vi "Settings Dialog.vi"(8 "error in (no error)":errorcluster, 11 "Settings in":T12={"Hardware Configuration"={"VISA resource name"="", "DAQ Type"=0, "Channel 1"={"Acquiring"=FALSE, "Enabled"=FALSE, "Terminal configuration"=32767, "Range"=0, "Coupling"=0}, "Channel 2"={"Acquiring"=FALSE, "Enabled"=FALSE, "Terminal configuration"=0, "Range"=0, "Coupling"=0}, "Timing"={"Sample Time [Time Units]"=0, "Actual Sample Time [s]"=0.0, "Samples per Iteration"=0, "Sample Clock Source"=0, "Time Units"=0, "t0"=timestamp(0 s since 1904-01-01)}, "PS Parameters"={"PS handle"=0, "PS Max_adc"=32767, "PS Enabled Array"=[], "PS Device Info"={"Driver Version"="", "USB Version"="", "Hardware"="", "Variant"="", "Batch and Serial"="", "Cal Date"="", "Kernel Version"="", "Digital HW Version"="", "Analogue HW Version"="", "Firmware 1"="", "Firmware 2"="", "MSO"=FALSE, "Number of Channels"=0}, "Channel 1 Buffer"=refnum, "Channel 2 Buffer"=refnum, "Resolution"=0, "USB Power"=FALSE}, "Trigger"={"Direction"=0, "Threshold [V]"=0.0, "Enabled"=FALSE, "Trigger Source"=0}, "Keithley Parameters"={"Previous End / Current Start"=0, "Quantity"=0}}, "Logging Configuration"={"Log File Base Path"=path "", "TDMS File Reference"=refnum, "Enabled"=FALSE, "Disk cache size"=0}} {"Hardware Configuration"."Keithley Parameters"."Quantity" items=["Current", "Voltage"]; "Hardware Configuration"."Trigger"."Trigger Source" items=["Channel 1"=0, "Channel 2"=1, "Ext."=4]; "Hardware Configuration"."Trigger"."Direction" items=["Falling", "Rising"]; "Hardware Configuration"."PS Parameters"."Resolution" items=["8", "12", "14", "15", "16"]; "Hardware Configuration"."Timing"."Time Units" items=["Seconds"]; "Hardware Configuration"."Timing"."Sample Clock Source" items=["Internal", "External"]; "Hardware Configuration"."Channel 2"."Coupling" items=["AC", "DC"]; "Hardware Configuration"."Channel 2"."Range" items=["0.01", "0.02", "0.05", "0.1", "0.2", "0.5", "1", "2", "5", "10", "20", "50", "100", "1000"]; "Hardware Configuration"."Channel 2"."Terminal configuration" items=["Referenced Single Ended", "Differential"]; "Hardware Configuration"."Channel 1"."Coupling" items=["AC", "DC"]; "Hardware Configuration"."Channel 1"."Range" items=["0.01", "0.02", "0.05", "0.1", "0.2", "0.5", "1", "2", "5", "10", "20", "50", "100", "1000"]; "Hardware Configuration"."Channel 1"."Terminal configuration" items=["Referenced Single Ended", "Differential"]; "Hardware Configuration"."DAQ Type" items=["Simulated", "Tektronics DPO2k/3k/4k", "PicoScope 2000a Series", "Keithley DMM7510", "PicoScope 5000a Series"]}) -> (0 "error out":errorcluster, 1 "Cancelled?":bool, 2 "UI Refresh Needed?":bool, 3 "Settings out":T12={"Hardware Configuration"={"VISA resource name"="", "DAQ Type"=0, "Channel 1"={"Acquiring"=FALSE, "Enabled"=FALSE, "Terminal configuration"=32767, "Range"=0, "Coupling"=0}, "Channel 2"={"Acquiring"=FALSE, "Enabled"=FALSE, "Terminal configuration"=0, "Range"=0, "Coupling"=0}, "Timing"={"Sample Time [Time Units]"=0, "Actual Sample Time [s]"=0.0, "Samples per Iteration"=0, "Sample Clock Source"=0, "Time Units"=0, "t0"=timestamp(0 s since 1904-01-01)}, "PS Parameters"={"PS handle"=0, "PS Max_adc"=32767, "PS Enabled Array"=[], "PS Device Info"={"Driver Version"="", "USB Version"="", "Hardware"="", "Variant"="", "Batch and Serial"="", "Cal Date"="", "Kernel Version"="", "Digital HW Version"="", "Analogue HW Version"="", "Firmware 1"="", "Firmware 2"="", "MSO"=FALSE, "Number of Channels"=0}, "Channel 1 Buffer"=refnum, "Channel 2 Buffer"=refnum, "Resolution"=0, "USB Power"=FALSE}, "Trigger"={"Direction"=0, "Threshold [V]"=0.0, "Enabled"=FALSE, "Trigger Source"=0}, "Keithley Parameters"={"Previous End / Current Start"=0, "Quantity"=0}}, "Logging Configuration"={"Log File Base Path"=path "", "TDMS File Reference"=refnum, "Enabled"=FALSE, "Disk cache size"=0}} {"Hardware Configuration"."Keithley Parameters"."Quantity" items=["Current", "Voltage"]; "Hardware Configuration"."Trigger"."Trigger Source" items=["Channel 1"=0, "Channel 2"=1, "Ext."=4]; "Hardware Configuration"."Trigger"."Direction" items=["Falling", "Rising"]; "Hardware Configuration"."PS Parameters"."Resolution" items=["8", "12", "14", "15", "16"]; "Hardware Configuration"."Timing"."Time Units" items=["Seconds"]; "Hardware Configuration"."Timing"."Sample Clock Source" items=["Internal", "External"]; "Hardware Configuration"."Channel 2"."Coupling" items=["AC", "DC"]; "Hardware Configuration"."Channel 2"."Range" items=["0.01", "0.02", "0.05", "0.1", "0.2", "0.5", "1", "2", "5", "10", "20", "50", "100", "1000"]; "Hardware Configuration"."Channel 2"."Terminal configuration" items=["Referenced Single Ended", "Differential"]; "Hardware Configuration"."Channel 1"."Coupling" items=["AC", "DC"]; "Hardware Configuration"."Channel 1"."Range" items=["0.01", "0.02", "0.05", "0.1", "0.2", "0.5", "1", "2", "5", "10", "20", "50", "100", "1000"]; "Hardware Configuration"."Channel 1"."Terminal configuration" items=["Referenced Single Ended", "Differential"]; "Hardware Configuration"."DAQ Type" items=["Simulated", "Tektronics DPO2k/3k/4k", "PicoScope 2000a Series", "Keithley DMM7510", "PicoScope 5000a Series"]})   [LabVIEW 2016, in "Settings.lvlib"]
doc: "Dialog for selecting user specified settings."
uses:
  Settings.lvlib
  Settings.ctl
  Acquisition/Hardware Configuration.ctl
  Acquisition/Signal Type.ctl
  Terminal Configuration.ctl
  Range.ctl
  Coupling.ctl
  Sampling Clock Source.ctl
  Time Units.ctl
  Resolution.ctl
  Trigger Direction.ctl
  Trigger Source.ctl
  Quantity.ctl
  Logging/Logging Configuration.ctl
  Physical Connection.ctl
  <vilib>/Utility/xml.llb/Write to XML File(string).vi
  Acquisition/Acquisition.lvlib
  Logging/Logging.lvlib
panel:
  in  "Quantity":T1=1 items=["Current", "Voltage"]
  in  "USB Powered":bool
  in  "Resolution":T2 items=["8", "12", "14", "15", "16"]
  in  "Coupling":T3=1 items=["AC", "DC"]
  in  "Coupling":T3=1 items=["AC", "DC"]
  in  "Time Unit":T4=4 items=["ns"=2, "us"=3, "ms"=4, "s"=5]
  in  "Tab Control":enum32{"Disabled", "Analog", "Digital"}(tab)
  in  "Direction":T5 items=["Either"=0, "Rising"=3, "Falling"=4]
  in  "Threshold [V]":dbl
  in  "Trigger Source":T6 items=["Channel 1"=0, "Channel 2"=1, "External"=4]
  in  "On/Off":bool=TRUE
  in  "Range":T7 items=["10 u"=50, "100 u"=51, "1 m"=52, "10 m"=0, "20 m"=1, "50 m"=2, "100 m"=3, "200 m"=4, "500 m"=5, "1"=6, "2"=7, "3"=53, "5"=8, "10"=9, "20"=10, "50"=11, "100"=12, "700"=90, "1000"=13]
  in  "Range":T7 items=["10 u"=50, "100 u"=51, "1 m"=52, "10 m"=0, "20 m"=1, "50 m"=2, "100 m"=3, "200 m"=4, "500 m"=5, "1"=6, "2"=7, "3"=53, "5"=8, "10"=9, "20"=10, "50"=11, "100"=12, "700"=90, "1000"=13]
  out "Samples per Iteration":dbl
  out "Actual Samping Time":dbl
  in  "Sampling Time":u32=1 min=1
  in  "Sampling Clock Source":T8 items=["Internal", "External"]
  out "Acquiring":bool
  out "Acquiring":bool
  in  "Terminal configuration":T9 items=["Referenced Single Ended", "Differential"]
  in  "Physical connection":T10 items=["Disabled", "Channel 1", "Channel 2"]
  in  "Terminal configuration":T9 items=["Referenced Single Ended", "Differential"]
  in  "Physical connection":T10 items=["Disabled", "Channel 1", "Channel 2"]
  in  "VISA resource name":refnum<visa-resource-name>
  in  "Log File Path":path
  in  "DAQ Type":T11 items=["Simulated", "Tektronics DPO2k/3k/4k", "PicoScope 2000a Series", "Keithley DMM7510", "PicoScope 5000a Series"]
  in  "Cancel Button":bool
  in  "OK Button":bool
  # "Non visible portion of dialog (needed for connector pane)."
  # "General Settings"
  # "Timing Settings"
  # "Channel Settings (Signal 1)"
  # "Trigger Settings"
  # "Channel Settings (Signal 2)"
  # "Logging"
  # "To configure and use a start trigger you must select\nthe specific tab. Not all hardware supports triggering.\nRefer to your device documentation for more info"
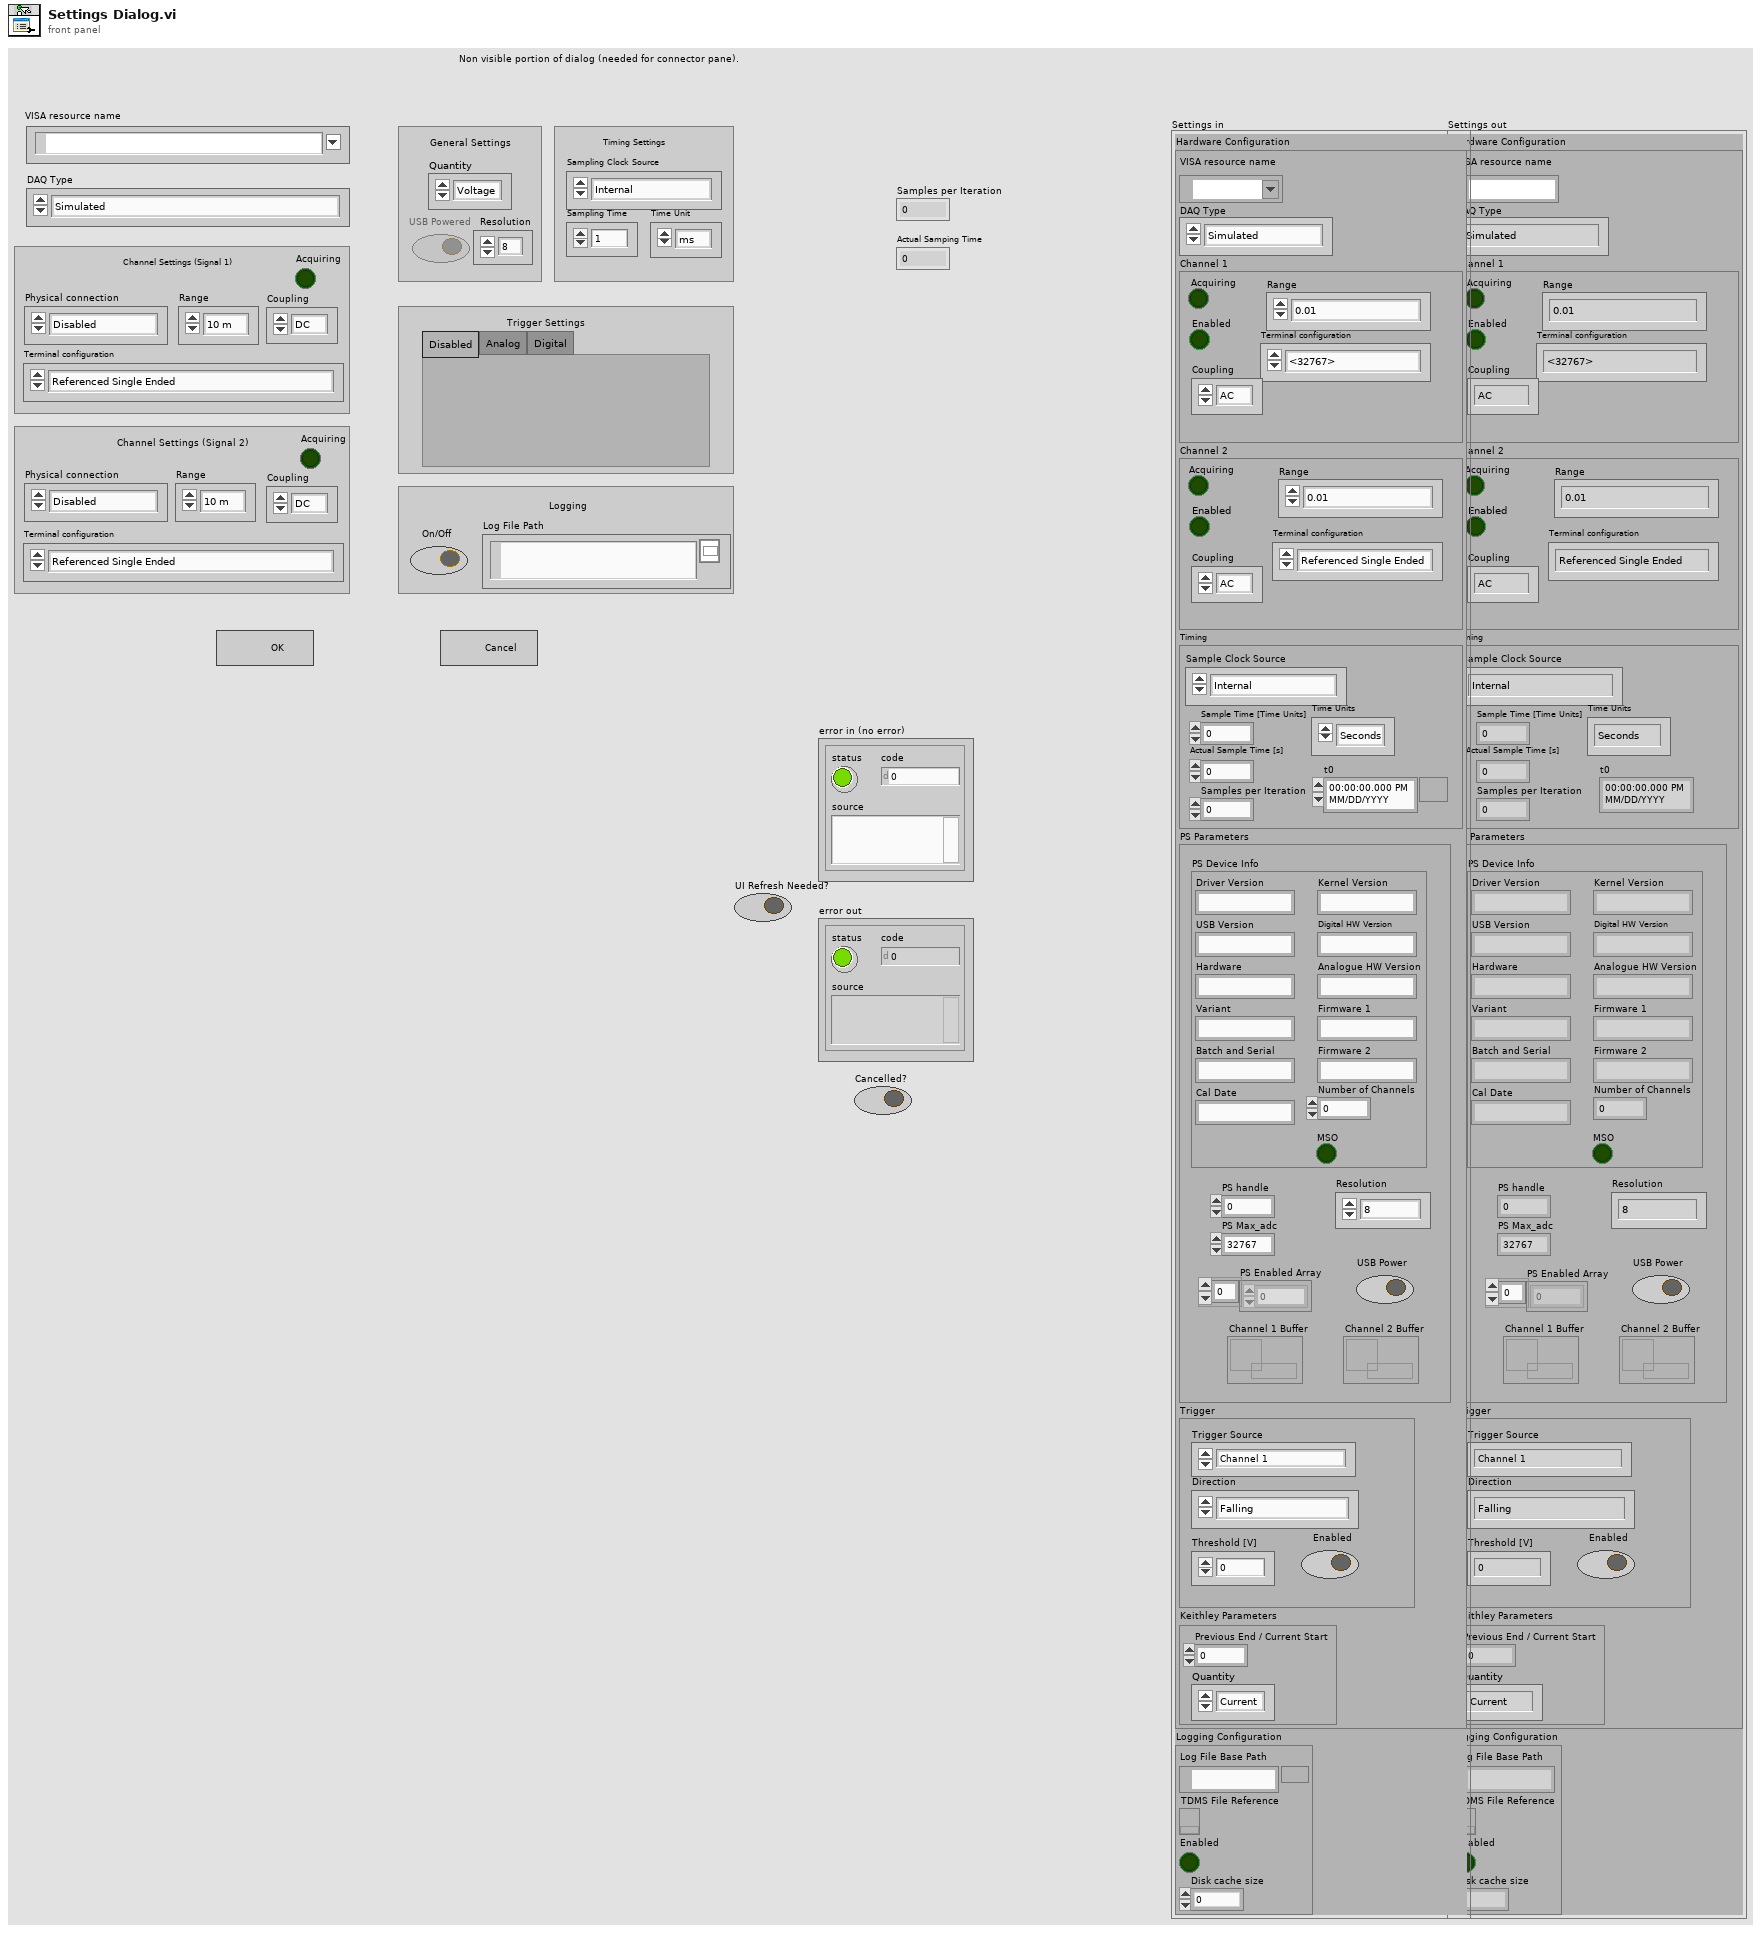
[diagram p1: front panel]
types:
  T1 = typedef "Settings.lvlib/Quantity.ctl" = u16
  T2 = typedef "Settings.lvlib/Resolution.ctl" = i32
  T3 = typedef "Settings.lvlib/Coupling.ctl" = i16
  T4 = typedef "Settings.lvlib/Time Units.ctl" = u32
  T5 = typedef "Settings.lvlib/Trigger Direction.ctl" = u16
  T6 = typedef "Settings.lvlib/Trigger Source.ctl" = u16
  T7 = typedef "Settings.lvlib/Range.ctl" = u16
  T8 = typedef "Settings.lvlib/Sampling Clock Source.ctl" = u16
  T9 = typedef "Settings.lvlib/Terminal Configuration.ctl" = u16
  T10 = typedef "Settings.lvlib/Physical Connection.ctl" = u16
  T11 = typedef "Acquisition.lvlib/Signal Type.ctl" = u16
  T12 = typedef "Settings.lvlib/Settings.ctl" = cluster{"Hardware Configuration":T13, "Logging Configuration":T14}
  T13 = typedef "Acquisition.lvlib/Hardware Configuration.ctl" = cluster{"VISA resource name":refnum<visa-resource-name>, "DAQ Type":T11, "Channel 1":cluster{"Acquiring":bool, "Enabled":bool, "Terminal configuration":T9, "Range":T7, "Coupling":T3}, "Channel 2":cluster{"Acquiring":bool, "Enabled":bool, "Terminal configuration":T9, "Range":T7, "Coupling":T3}, "Timing":cluster{"Sample Time [Time Units]":u32, "Actual Sample Time [s]":dbl, "Samples per Iteration":u32, "Sample Clock Source":T8, "Time Units":T4, "t0":timestamp}, "PS Parameters":cluster{"PS handle":i16, "PS Max_adc":i16, "PS Enabled Array":i16[], "PS Device Info":cluster{"Driver Version":string, "USB Version":string, "Hardware":string, "Variant":string, "Batch and Serial":string, "Cal Date":string, "Kernel Version":string, "Digital HW Version":string, "Analogue HW Version":string, "Firmware 1":string, "Firmware 2":string, "MSO":bool, "Number of Channels":i16}, "Channel 1 Buffer":refnum<data-value>, "Channel 2 Buffer":refnum<data-value>, "Resolution":T2, "USB Power":bool}, "Trigger":cluster{"Direction":T5, "Threshold [V]":dbl, "Enabled":bool, "Trigger Source":T6}, "Keithley Parameters":cluster{"Previous End / Current Start":i32, "Quantity":T1}}
  T14 = typedef "Logging.lvlib/Logging Configuration.ctl" = cluster{"Log File Base Path":path, "TDMS File Reference":refnum<k34>, "Enabled":bool, "Disk cache size":u64}
  T15 = enum8{"Enabled", "Disabled", "Disabled and Grayed Out"}
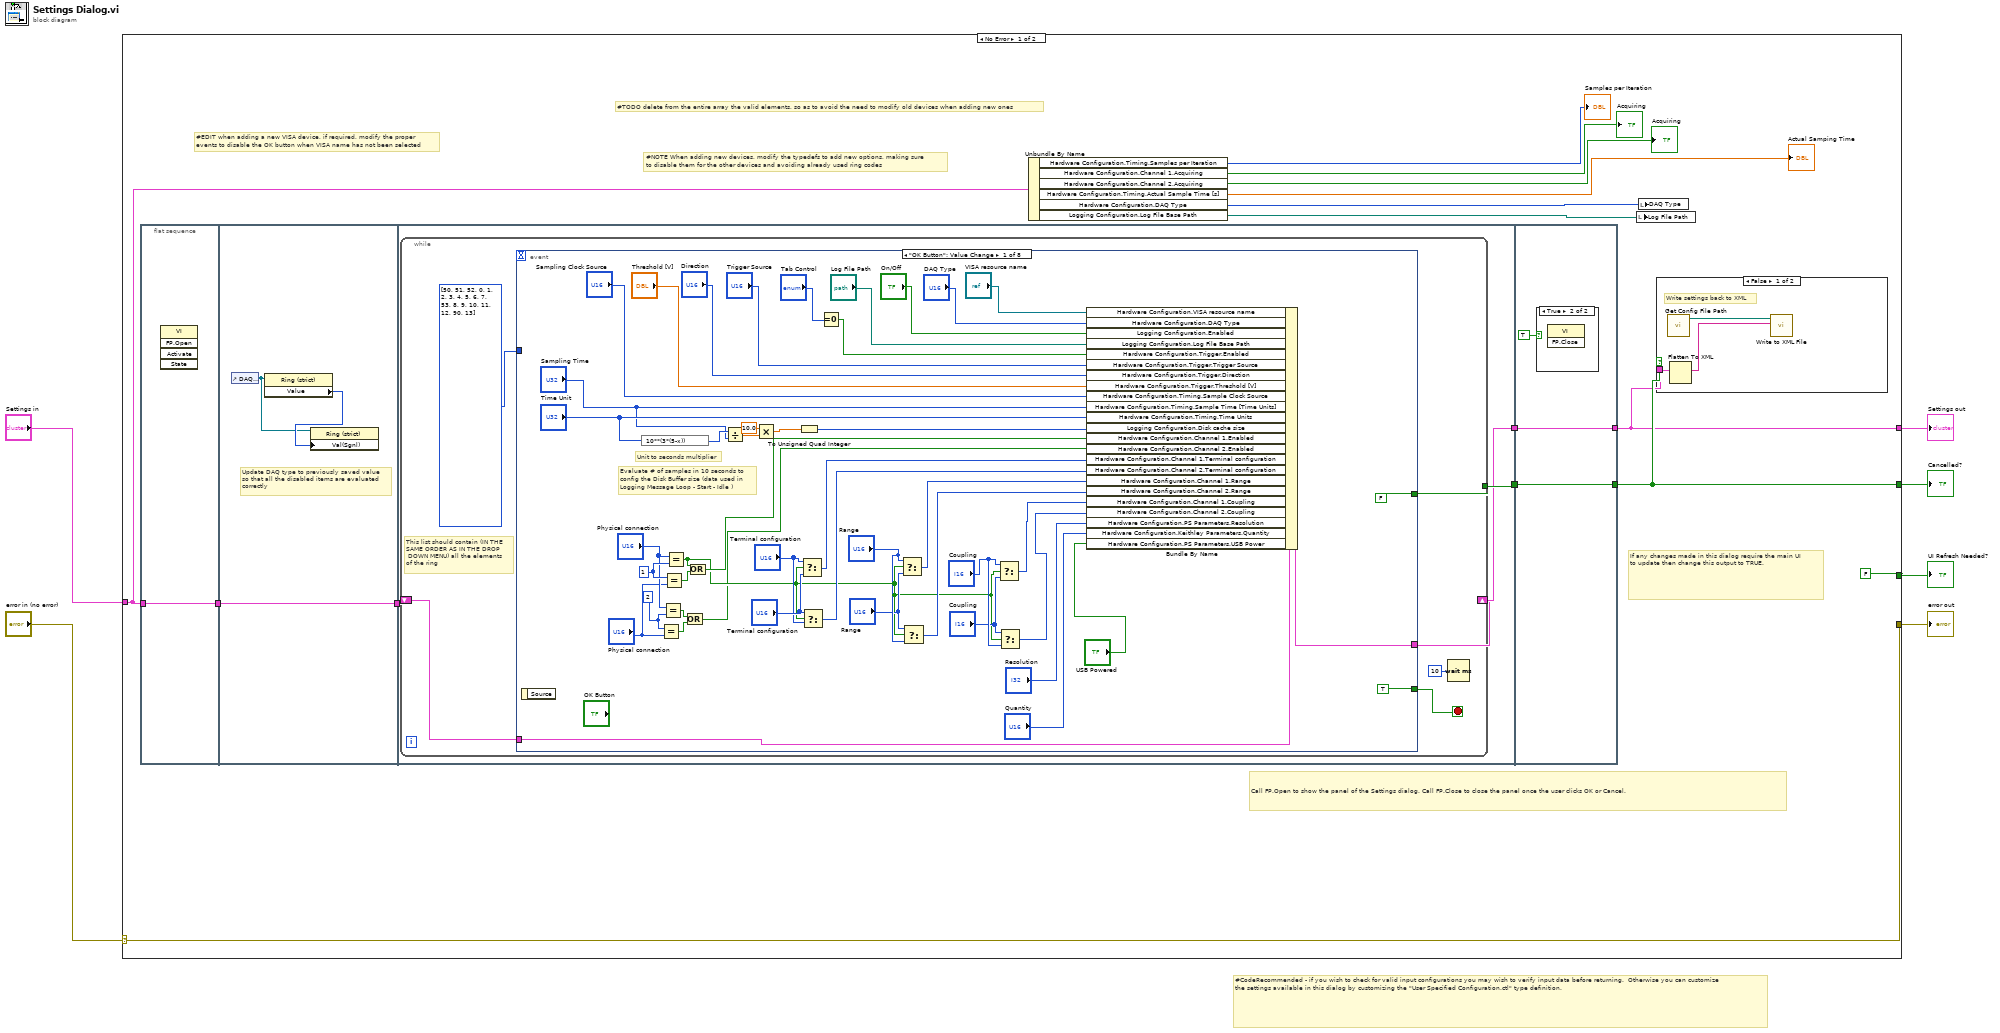
[diagram p0: block diagram]
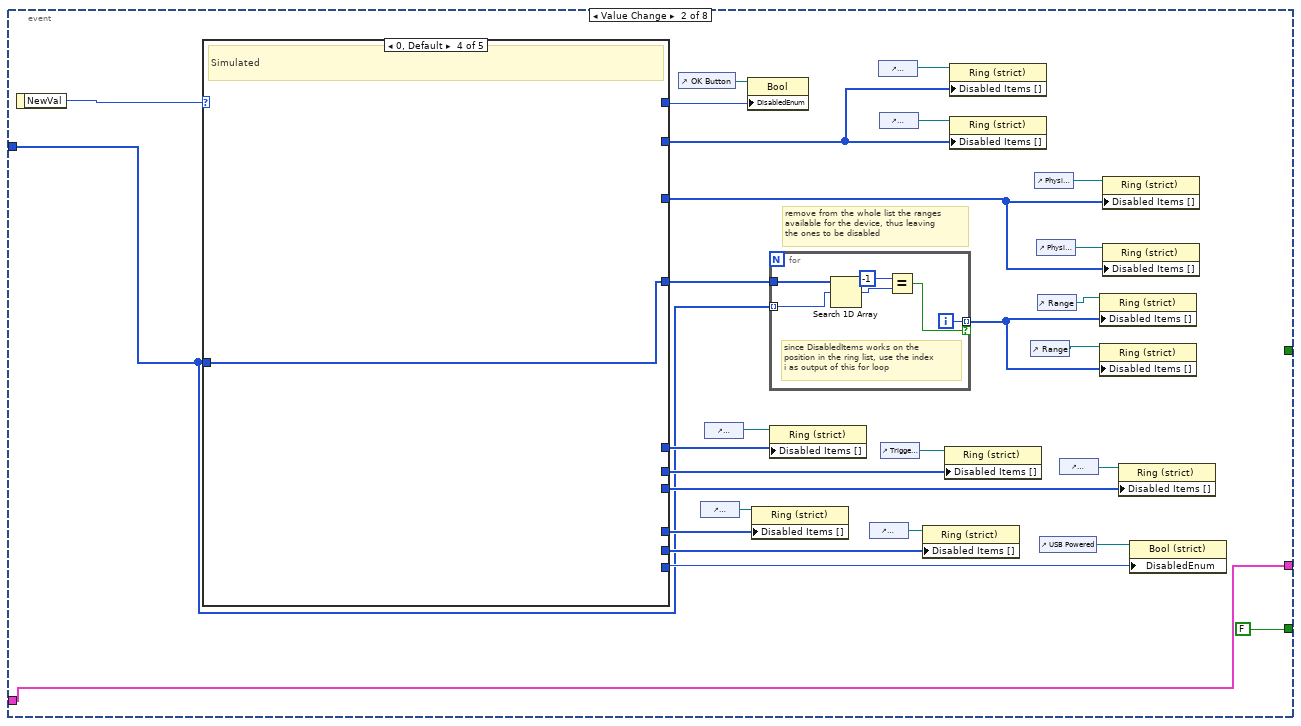
[diagram p2: hidden frame]
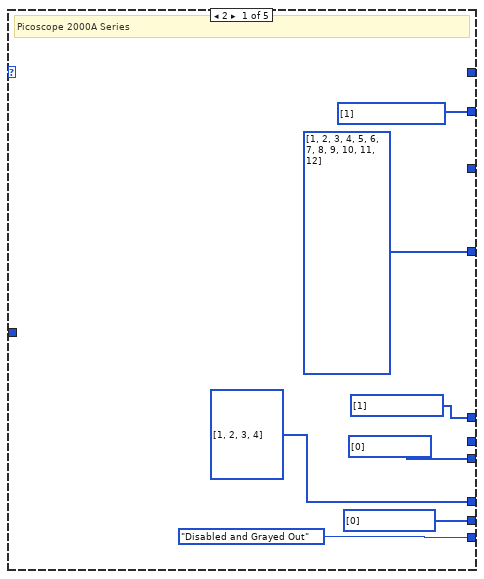
[diagram p3: hidden frame]
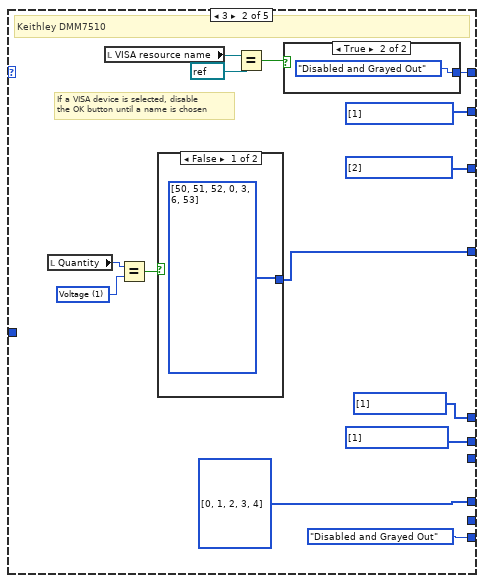
[diagram p4: hidden frame]
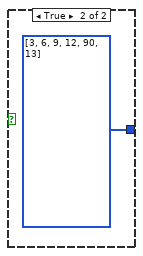
[diagram p5: hidden frame]
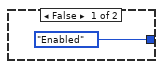
[diagram p6: hidden frame]
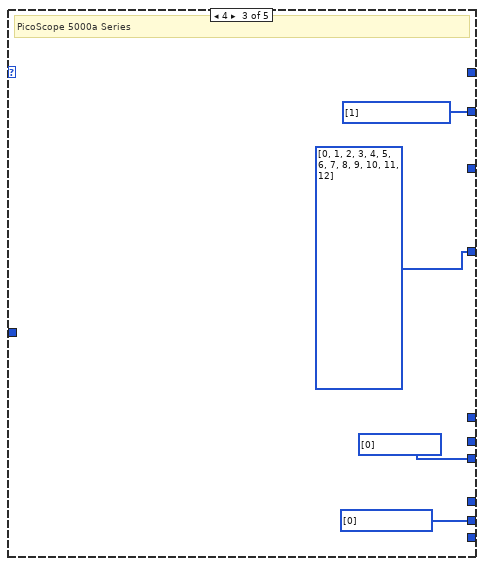
[diagram p7: hidden frame]
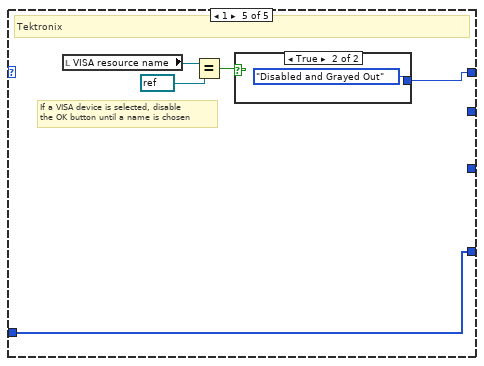
[diagram p8: hidden frame]
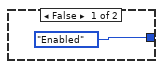
[diagram p9: hidden frame]
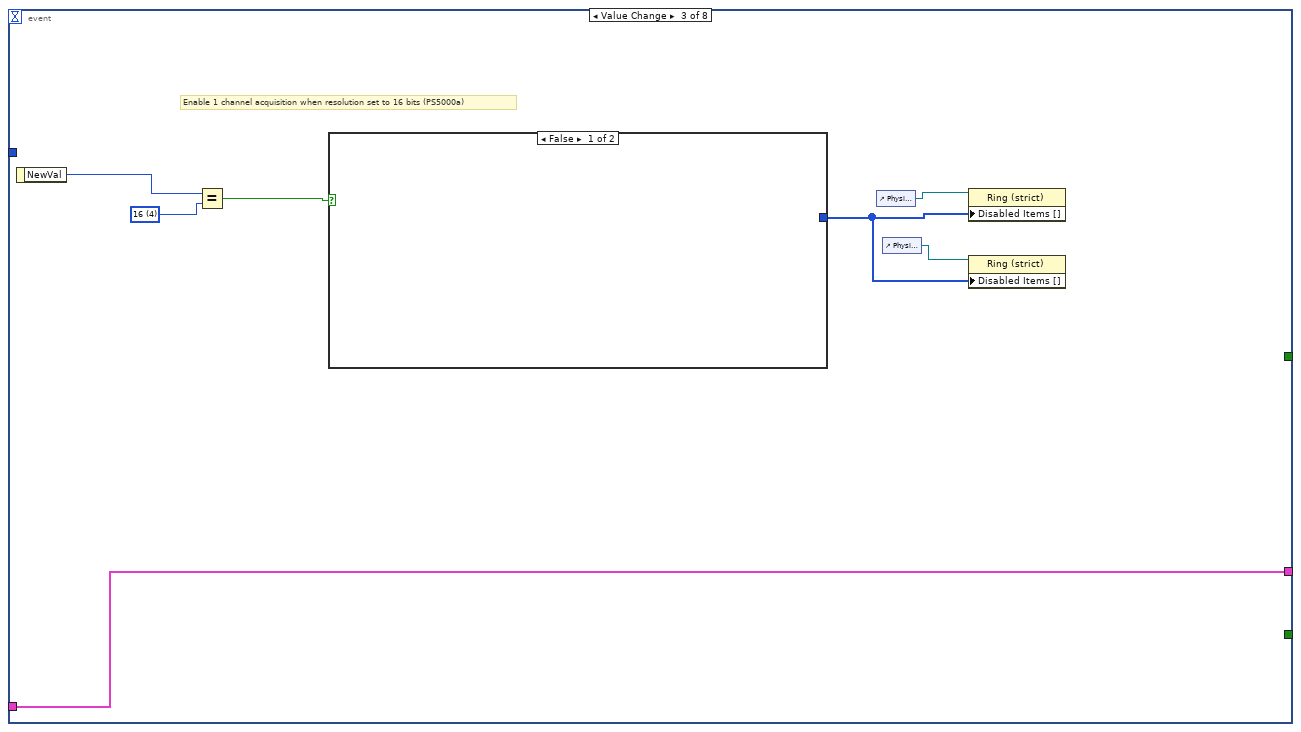
[diagram p10: hidden frame]
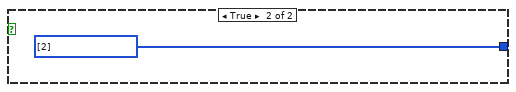
[diagram p11: hidden frame]
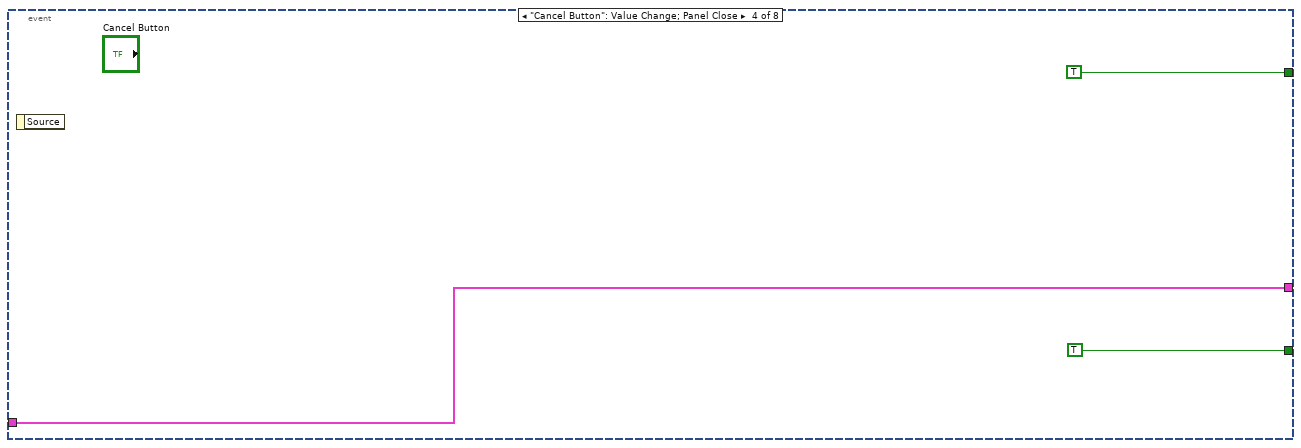
[diagram p12: hidden frame]
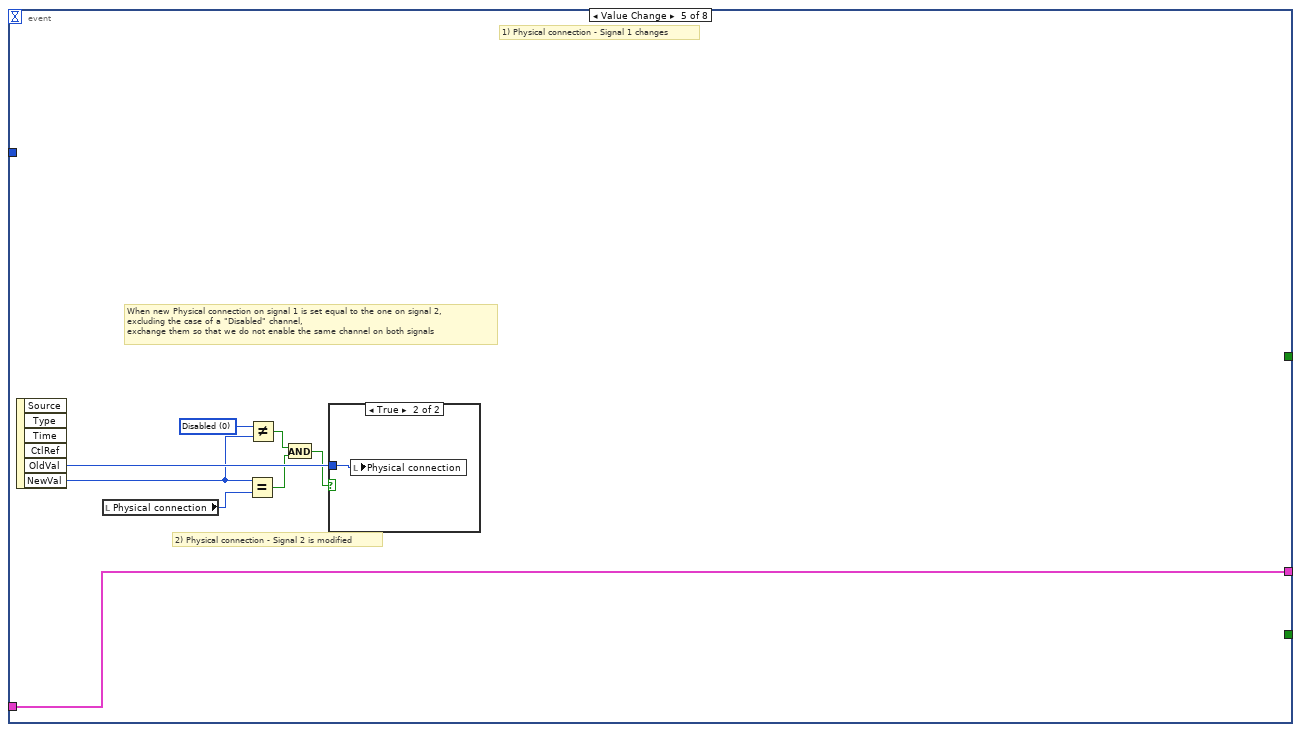
[diagram p13: hidden frame]
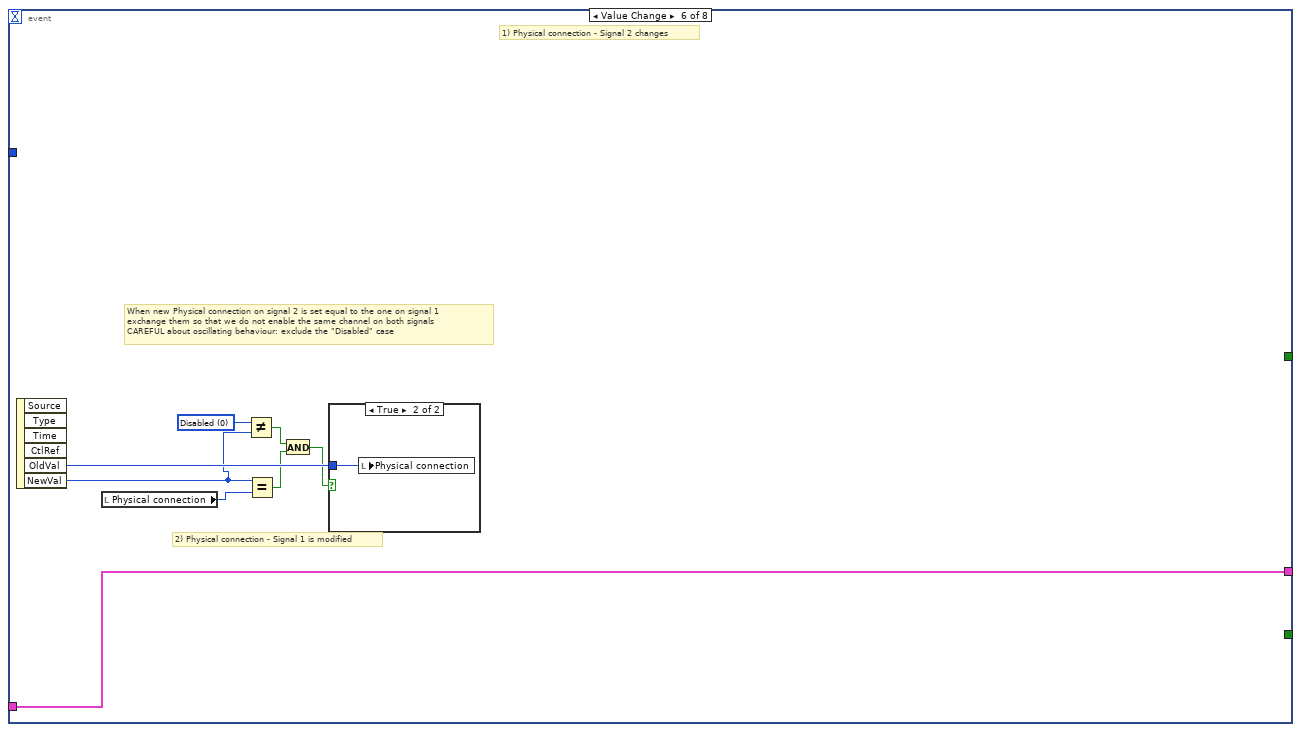
[diagram p15: hidden frame]
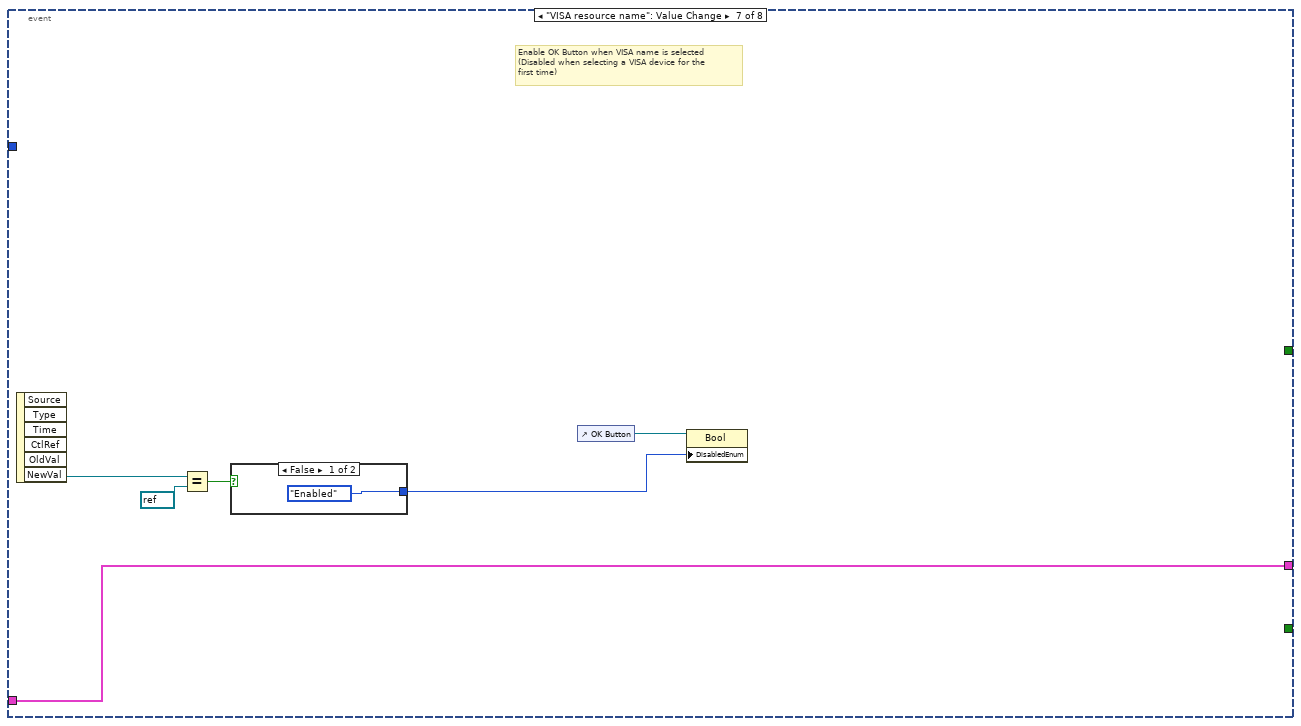
[diagram p17: hidden frame]
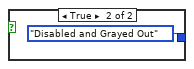
[diagram p18: hidden frame]
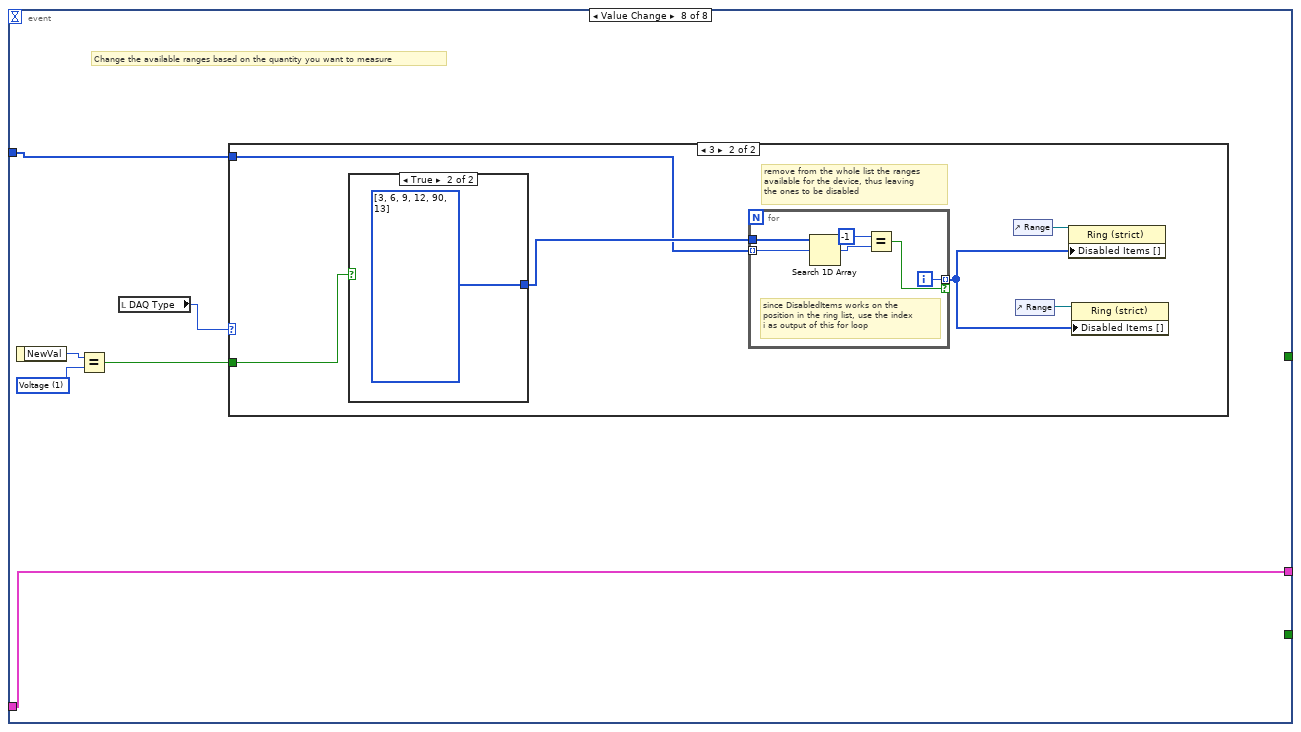
[diagram p19: hidden frame]
diagram:
  # "#CodeRecommended - if you wish to check for valid input configurations you may wish to verify input data before returning.  Otherwise you can customize the settings available in this dialog by customizing the \"User Specified Configuration.ctl\" type definition."
  n1 = case shown="No Error" "error in (no error)" {
    selector: "error in (no error)" -> [w21 w217]
    tunnel: [w21 w217] -> w5
    tunnel: "Settings in" -> [w17 w216]
    tunnel: [w18 w216] -> w3
    tunnel: [FALSE ("UI Refresh Needed?") _] -> w2
    tunnel: [w19 TRUE ("UI Refresh Needed?")] -> w1
    frame No Error {
      # "#EDIT when adding a new VISA device, if required, modify the proper\nevents to disable the OK button when VISA name has not been selected"
      # "#TODO delete from the entire array the valid elements, so as to avoid the need to modify old devices when adding new ones"
      # "#NOTE When adding new devices, modify the typedefs to add new options, making sure\nto disable them for the other devices and avoiding already used ring codes"
      # "Call FP.Open to show the panel of the Settings dialog. Call FP.Close to close the panel once the user clicks OK or Cancel."
      # "If any changes made in this dialog require the main UI to update then change this output to TRUE."
      n2 = flat-sequence {
        tunnel: w17 -> [w22]
        tunnel: [w22] -> w8
        tunnel: w8 -> [w25]
        tunnel: [w25] -> w7
        tunnel: w7 -> [w26]
        tunnel: [w28] -> w14
        tunnel: [w27] -> w13
        tunnel: [w210] -> w18
        tunnel: [w211] -> w19
        tunnel: w14 -> [w211]
        tunnel: w13 -> [w210]
        frame #0 {
          n3 = invoke class="VI" method="FP.Open"() -> ()  [unwired: 5 in, 5 out]
        }
        frame #1 {
          # "Update DAQ type to previously saved value\nso that all the disabled items are evaluated\ncorrectly"
          n4 = control-ref of="DAQ Type"() -> (w23:refnum<vi>)
          n5 = property class="Ring (strict)"(reference=w23) -> ("Value"=w24:T11)  [unwired: 1 in, 2 out]
          n6 = property class="Ring (strict)"(reference=w23, "Val(Sgnl)"=w24) -> ()  [unwired: 1 in, 2 out]
        }
        frame #2 {
          n7 = while {
            tunnel: [w34] -> w28
            shift-right: [w33] -> w27
            shift-left: w26 -> [w32]
            stop <- w31 stop-if-true
            w29 = T7[] [50, 51, 52, 0, 1, 2, 3, 4, 5, 6, 7, 53, 8, 9, 10, 11, 12, 90, 13] items=["10 u"=50, "100 u"=51, "1 m"=52, "10 m"=0, "20 m"=1, "50 m"=2, "100 m"=3, "200 m"=4, "500 m"=5, "1"=6, "2"=7, "3"=53, "5"=8, "10"=9, "20"=10, "50"=11, "100"=12, "700"=90, "1000"=13] ("Range [V]")
            # "This list should contain (IN THE \nSAME ORDER AS IN THE DROP\n DOWN MENU) all the elements \nof the ring"
            n8 = event shown="[0] \"OK Button\": Value Change" {
              selector: _ -> [_ _ _ _ _ _ _ _]
              dyn-events: _ -> [_ _ _ _ _ _ _ _]
              timeout: _ -> [_ _ _ _ _ _ _ _]
              tunnel: [w78 w108 w158 w162 w170 w179 w186 w194] -> w33
              tunnel: w32 -> [w79 w108 w158 w162 w170 w179 w186 w194]
              tunnel: [FALSE ("UI Refresh Needed?") _ _ TRUE ("UI Refresh Needed?") _ _ _ _] -> w34
              tunnel: [TRUE FALSE _ TRUE _ _ _ _] -> w31
              tunnel: w29 -> [_ w81 _ _ _ _ _ w189]
              event "OK Button": Value Change {
                w71 = u16 2 ("x")
                w73 = u16 1 ("x")
                # "Evaluate # of samples in 10 seconds to \nconfig the Disk Buffer size (data used in \nLogging Message Loop - Start - Idle )"
                # "Unit to seconds multiplier"
                n9 = event-data() -> ()  [unwired: 1 in, 1 out]
                n10 = expression code="10**(3*(5-x))"("Time Unit") -> (w40:T4)
                n11 = Equal?(x=w71, y="Physical connection") -> (x = y?=w70:bool)
                n12 = Equal?(x="Physical connection", y=w71) -> (x = y?=w62:bool)
                n13 = Equal?(x=w73, y="Physical connection") -> (x = y?=w72:bool)
                n14 = Equal?(x="Physical connection", y=w73) -> (x = y?=w49:bool)
                n15 = Or(x=w62, y=w70) -> (x .or. y?=w48:bool)
                n16 = Or(x=w49, y=w72) -> (x .or. y?=w59:bool)
                n17 = Divide(x=w40, y="Sampling Time") -> (x/y=w38:dbl)
                n18 = Multiply(x=10.0, y=w38) -> (x*y=w36:dbl)
                n19 = To Unsigned Quad Integer(1:w36) -> (0:w35:u64)
                n20 = Select(t="Terminal configuration", s=w49, f="Terminal configuration") -> (s? t:f=w47:T9)
                n21 = Select(t="Terminal configuration", s=w49, f="Terminal configuration") -> (s? t:f=w65:T9)
                n22 = Equal To 0?(x="Tab Control") -> (x = 0?=w57:bool)
                n23 = Select(t="Range", s=w49, f="Range") -> (s? t:f=w61:T7)
                n24 = Select(t="Range", s=w49, f="Range") -> (s? t:f=w53:T7)
                n25 = Select(t="Coupling", s=w49, f="Coupling") -> (s? t:f=w46:T3)
                n26 = Select(t="Coupling", s=w49, f="Coupling") -> (s? t:f=w45:T3)
                n27 = Bundle By Name(cluster=w79, "Hardware Configuration.VISA resource name"="VISA resource name", "Hardware Configuration.DAQ Type"="DAQ Type", "Logging Configuration.Enabled"="On/Off", "Logging Configuration.Log File Base Path"="Log File Path", "Hardware Configuration.Trigger.Enabled"=w57, "Hardware Configuration.Trigger.Trigger Source"="Trigger Source", "Hardware Configuration.Trigger.Direction"="Direction", "Hardware Configuration.Trigger.Threshold [V]"="Threshold [V]", "Hardware Configuration.Timing.Sample Clock Source"="Sampling Clock Source", "Hardware Configuration.Timing.Sample Time [Time Units]"="Sampling Time", "Hardware Configuration.Timing.Time Units"="Time Unit", "Logging Configuration.Disk cache size"=w35, "Hardware Configuration.Channel 1.Enabled"=w59, "Hardware Configuration.Channel 2.Enabled"=w48, "Hardware Configuration.Channel 1.Terminal configuration"=w47, "Hardware Configuration.Channel 2.Terminal configuration"=w65, "Hardware Configuration.Channel 1.Range"=w61, "Hardware Configuration.Channel 2.Range"=w53, "Hardware Configuration.Channel 1.Coupling"=w46, "Hardware Configuration.Channel 2.Coupling"=w45, "Hardware Configuration.PS Parameters.Resolution"="Resolution", "Hardware Configuration.Keithley Parameters.Quantity"="Quantity", "Hardware Configuration.PS Parameters.USB Power"="USB Powered") -> (w78:T12)
              }
              event Value Change {
                # "remove from the whole list the ranges\navailable for the device, thus leaving \nthe ones to be disabled"
                n28 = event-data() -> ("NewVal"=w107:T11)  [unwired: 1 in]
                n29 = case shown="0, Default" w107 {
                  tunnel: [w121 w135 w143 _ _] -> w103
                  tunnel: [_ w134 _ _ _] -> w100
                  tunnel: [w120 w133 _ _ _] -> w98
                  tunnel: [_ w132 _ _ _] -> w96
                  tunnel: [w119 _ w142 _ _] -> w94
                  tunnel: [w118 w131 _ _ _] -> w92
                  tunnel: [w117 _ w141 _ _] -> w90
                  tunnel: [T15."Disabled and Grayed Out" ("Disabled") T15."Disabled and Grayed Out" ("Disabled") _ _ _] -> w88
                  tunnel: [_ w126 _ _ w146] -> w84
                  tunnel: [w115 w122 w140 w144 w145] -> w82
                  tunnel: w81 -> [_ _ _ w144 w145]
                  frame 2 {
                    w115 = T7[] [1, 2, 3, 4, 5, 6, 7, 8, 9, 10, 11, 12] items=["10 u"=50, "100 u"=51, "1 m"=52, "10 m"=0, "20 m"=1, "50 m"=2, "100 m"=3, "200 m"=4, "500 m"=5, "1"=6, "2"=7, "3"=53, "5"=8, "10"=9, "20"=10, "50"=11, "100"=12, "700"=90, "1000"=13] ("Disabled Items []")
                    w117 = T1[] [0] items=["Current", "Voltage"] ("Disabled Items []")
                    w118 = T2[] [1, 2, 3, 4] items=["8", "12", "14", "15", "16"] ("Disabled Items []")
                    w119 = u16[] [0] items=["Either"=0, "Rising"=3, "Falling"=4] ("Disabled Items []")
                    w120 = u16[] [1] items=["Internal", "External"] ("Disabled Items []")
                    w121 = T9[] [1] items=["Referenced Single Ended", "Differential"] ("Disabled Items []")
                    # "Picoscope 2000A Series"
                  }
                  frame 3 {
                    w124 = T1 1 items=["Current", "Voltage"] ("y")
                    w131 = T2[] [0, 1, 2, 3, 4] items=["8", "12", "14", "15", "16"] ("Disabled Items []")
                    w132 = u16[] [1] items=["Channel 1"=0, "Channel 2"=1, "External"=4] ("Disabled Items []")
                    w133 = u16[] [1] items=["Internal", "External"] ("Disabled Items []")
                    w134 = T10[] [2] items=["Disabled", "Channel 1", "Channel 2"] ("Disabled Items []")
                    w135 = T9[] [1] items=["Referenced Single Ended", "Differential"] ("Disabled Items []")
                    # "If a VISA device is selected, disable\nthe OK button until a name is chosen"
                    # "Keithley DMM7510"
                    n30 = local read "Quantity"() -> (w123:T1)
                    n31 = local read "VISA resource name"() -> (w129:refnum<visa-resource-name>)
                    n32 = Equal?(x=w123, y=w124) -> (x = y?=w125:bool)
                    n33 = case shown="False" w125 {
                      tunnel: [w136 w137] -> w122
                      frame False {
                        w136 = T7[] [50, 51, 52, 0, 3, 6, 53] items=["10 u"=50, "100 u"=51, "1 m"=52, "10 m"=0, "20 m"=1, "50 m"=2, "100 m"=3, "200 m"=4, "500 m"=5, "1"=6, "2"=7, "3"=53, "5"=8, "10"=9, "20"=10, "50"=11, "100"=12, "700"=90, "1000"=13] ("Range [V]")
                      }
                      frame True {
                        w137 = T7[] [3, 6, 9, 12, 90, 13] items=["10 u"=50, "100 u"=51, "1 m"=52, "10 m"=0, "20 m"=1, "50 m"=2, "100 m"=3, "200 m"=4, "500 m"=5, "1"=6, "2"=7, "3"=53, "5"=8, "10"=9, "20"=10, "50"=11, "100"=12, "700"=90, "1000"=13] ("Range [V]")
                      }
                    }
                    n34 = Equal?(x=w129, y=refnum<visa-resource-name> refnum) -> (x = y?=w127:bool)
                    n35 = case shown="True" w127 {
                      tunnel: [T15."Enabled" ("Disabled") T15."Disabled and Grayed Out" ("Disabled")] -> w126
                      frame False {
                      }
                      frame True {
                      }
                    }
                  }
                  frame 4 {
                    w140 = T7[] [0, 1, 2, 3, 4, 5, 6, 7, 8, 9, 10, 11, 12] items=["10 u"=50, "100 u"=51, "1 m"=52, "10 m"=0, "20 m"=1, "50 m"=2, "100 m"=3, "200 m"=4, "500 m"=5, "1"=6, "2"=7, "3"=53, "5"=8, "10"=9, "20"=10, "50"=11, "100"=12, "700"=90, "1000"=13] ("Disabled Items []")
                    w141 = T1[] [0] items=["Current", "Voltage"] ("Disabled Items []")
                    w142 = T5[] [0] items=["Either"=0, "Rising"=3, "Falling"=4] ("Disabled Items []")
                    w143 = T9[] [1] items=["Referenced Single Ended", "Differential"] ("Disabled Items []")
                    # "PicoScope 5000a Series"
                  }
                  frame 0, Default {
                    # "Simulated"
                  }
                  frame 1 {
                    # "If a VISA device is selected, disable\nthe OK button until a name is chosen"
                    # "Tektronix"
                    n36 = local read "VISA resource name"() -> (w149:refnum<visa-resource-name>)
                    n37 = Equal?(x=w149, y=refnum<visa-resource-name> refnum) -> (x = y?=w147:bool)
                    n38 = case shown="True" w147 {
                      tunnel: [T15."Enabled" ("Disabled") T15."Disabled and Grayed Out" ("Disabled")] -> w146
                      frame False {
                      }
                      frame True {
                      }
                    }
                  }
                }
                n39 = control-ref of="OK Button"() -> (w85:refnum<vi>)
                n40 = control-ref of="Resolution"() -> (w93:refnum<vi>)
                n41 = control-ref of="Sampling Clock Source"() -> (w99:refnum<vi>)
                n42 = property class="Bool"(reference=w85, "DisabledEnum"=w84) -> ()  [unwired: 1 in, 2 out]
                n43 = property class="Ring (strict)"(reference=w93, "Disabled Items []"=w92) -> ()  [unwired: 1 in, 2 out]
                n44 = for {
                  tunnel: [w112] -> w83 mode=indexing if=w111
                  tunnel: w82 -> [w110]
                  tunnel: w81 -> [w109] mode=indexing
                  i -> [w112]
                  # "since DisabledItems works on the\nposition in the ring list, use the index\ni as output of this for loop"
                  n45 = Search 1D Array(1D array=w110, element=w109) -> (index of element=w114:i32)  [unwired: 1 in]
                  n46 = Equal?(x=-1, y=w114) -> (x = y?=w111:bool)
                }
                n47 = property class="Ring (strict)"(reference=w99, "Disabled Items []"=w98) -> ()  [unwired: 1 in, 2 out]
                n48 = control-ref of="Quantity"() -> (w91:refnum<vi>)
                n49 = control-ref of="Terminal configuration"() -> (w105:refnum<vi>)
                n50 = control-ref of="Terminal configuration"() -> (w104:refnum<vi>)
                n51 = control-ref of="Trigger Source"() -> (w97:refnum<vi>)
                n52 = property class="Ring (strict)"(reference=w91, "Disabled Items []"=w90) -> ()  [unwired: 1 in, 2 out]
                n53 = property class="Ring (strict)"(reference=w97, "Disabled Items []"=w96) -> ()  [unwired: 1 in, 2 out]
                n54 = property class="Ring (strict)"(reference=w105, "Disabled Items []"=w103) -> ()  [unwired: 1 in, 2 out]
                n55 = property class="Ring (strict)"(reference=w104, "Disabled Items []"=w103) -> ()  [unwired: 1 in, 2 out]
                n56 = control-ref of="Range"() -> (w86:refnum<vi>)
                n57 = control-ref of="Physical connection"() -> (w102:refnum<vi>)
                n58 = control-ref of="Physical connection"() -> (w101:refnum<vi>)
                n59 = control-ref of="Range"() -> (w87:refnum<vi>)
                n60 = control-ref of="USB Powered"() -> (w89:refnum<vi>)
                n61 = control-ref of="Direction"() -> (w95:refnum<vi>)
                n62 = property class="Ring (strict)"(reference=w87, "Disabled Items []"=w83) -> ()  [unwired: 1 in, 2 out]
                n63 = property class="Ring (strict)"(reference=w86, "Disabled Items []"=w83) -> ()  [unwired: 1 in, 2 out]
                n64 = property class="Ring (strict)"(reference=w102, "Disabled Items []"=w100) -> ()  [unwired: 1 in, 2 out]
                n65 = property class="Ring (strict)"(reference=w101, "Disabled Items []"=w100) -> ()  [unwired: 1 in, 2 out]
                n66 = property class="Ring (strict)"(reference=w95, "Disabled Items []"=w94) -> ()  [unwired: 1 in, 2 out]
                n67 = property class="Bool (strict)"(reference=w89, "DisabledEnum"=w88) -> ()  [unwired: 1 in, 2 out]
              }
              event Value Change {
                w156 = T2 4 items=["8", "12", "14", "15", "16"] ("NewVal")
                # "Enable 1 channel acquisition when resolution set to 16 bits (PS5000a)"
                n68 = event-data() -> ("NewVal"=w157:T2)  [unwired: 1 in]
                n69 = Equal?(x=w157, y=w156) -> (x = y?=w155:bool)
                n70 = case shown="False" w155 {
                  tunnel: [_ w159] -> w152
                  frame False {
                  }
                  frame True {
                    w159 = T10[] [2] items=["Disabled", "Channel 1", "Channel 2"] ("Disabled Items []")
                  }
                }
                n71 = control-ref of="Physical connection"() -> (w153:refnum<vi>)
                n72 = control-ref of="Physical connection"() -> (w154:refnum<vi>)
                n73 = property class="Ring (strict)"(reference=w153, "Disabled Items []"=w152) -> ()  [unwired: 1 in, 2 out]
                n74 = property class="Ring (strict)"(reference=w154, "Disabled Items []"=w152) -> ()  [unwired: 1 in, 2 out]
              }
              event "Cancel Button": Value Change; Panel Close {
                n75 = event-data() -> ()  [unwired: 1 in, 1 out]
              }
              event Value Change {
                w166 = T10 0 items=["Disabled", "Channel 1", "Channel 2"] ("x")
                # "2) Physical connection - Signal 2 is modified"
                # "1) Physical connection - Signal 1 changes"
                # "When new Physical connection on signal 1 is set equal to the one on signal 2,\nexcluding the case of a \"Disabled\" channel, \nexchange them so that we do not enable the same channel on both signals"
                n76 = event-data() -> ("OldVal"=w168:T10, "NewVal"=w167:T10)  [unwired: 1 in, 4 out]
                n77 = local read "Physical connection"() -> (w169:T10)
                n78 = Equal?(x=w167, y=w169) -> (x = y?=w164:bool)
                n79 = Not Equal?(x=w166, y=w167) -> (x != y?=w165:bool)
                n80 = And(x=w165, y=w164) -> (x .and. y?=w163:bool)
                n81 = case shown="True" w163 {
                  tunnel: w168 -> [_ w171]
                  frame False {
                  }
                  frame True {
                    n82 = local write "Physical connection"(w171) -> ()
                  }
                }
              }
              event Value Change {
                w176 = T10 0 items=["Disabled", "Channel 1", "Channel 2"] ("x")
                # "2) Physical connection - Signal 1 is modified"
                # "1) Physical connection - Signal 2 changes"
                # "When new Physical connection on signal 2 is set equal to the one on signal 1\nexchange them so that we do not enable the same channel on both signals\nCAREFUL about oscillating behaviour: exclude the \"Disabled\" case"
                n83 = event-data() -> ("OldVal"=w178:T10, "NewVal"=w172:T10)  [unwired: 1 in, 4 out]
                n84 = local read "Physical connection"() -> (w177:T10)
                n85 = Not Equal?(x=w176, y=w172) -> (x != y?=w175:bool)
                n86 = Equal?(x=w172, y=w177) -> (x = y?=w173:bool)
                n87 = And(x=w175, y=w173) -> (x .and. y?=w174:bool)
                n88 = case shown="True" w174 {
                  tunnel: w178 -> [_ w180]
                  frame False {
                  }
                  frame True {
                    n89 = local write "Physical connection"(w180) -> ()
                  }
                }
              }
              event "VISA resource name": Value Change {
                # "Enable OK Button when VISA name is selected\n(Disabled when selecting a VISA device for the\nfirst time)"
                n90 = event-data() -> ("NewVal"=w185:refnum<visa-resource-name>)  [unwired: 1 in, 5 out]
                n91 = Equal?(x=w185, y=refnum<visa-resource-name> refnum) -> (x = y?=w182:bool)
                n92 = case shown="False" w182 {
                  tunnel: [T15."Enabled" ("Disabled") T15."Disabled and Grayed Out" ("Disabled")] -> w181
                  frame False {
                  }
                  frame True {
                  }
                }
                n93 = control-ref of="OK Button"() -> (w183:refnum<vi>)
                n94 = property class="Bool"(reference=w183, "DisabledEnum"=w181) -> ()  [unwired: 1 in, 2 out]
              }
              event Value Change {
                w192 = T1 1 items=["Current", "Voltage"] ("y")
                # "Change the available ranges based on the quantity you want to measure"
                n95 = event-data() -> ("NewVal"=w193:T1)  [unwired: 1 in]
                n96 = Equal?(x=w193, y=w192) -> (x = y?=w191:bool)
                n97 = local read "DAQ Type"() -> (w190:T11)
                n98 = case shown="3" w190 {
                  tunnel: w191 -> [_ w200]
                  tunnel: w189 -> [_ w195]
                  frame 0, Default {
                    # "Do nothing for the other devices so as not to enable unusable ranges"
                  }
                  frame 3 {
                    # "remove from the whole list the ranges\navailable for the device, thus leaving \nthe ones to be disabled"
                    n99 = case shown="True" w200 {
                      tunnel: [w207 w208] -> w196
                      frame False {
                        w207 = T7[] [50, 51, 52, 0, 3, 6, 53] items=["10 u"=50, "100 u"=51, "1 m"=52, "10 m"=0, "20 m"=1, "50 m"=2, "100 m"=3, "200 m"=4, "500 m"=5, "1"=6, "2"=7, "3"=53, "5"=8, "10"=9, "20"=10, "50"=11, "100"=12, "700"=90, "1000"=13] ("Range [V]")
                      }
                      frame True {
                        w208 = T7[] [3, 6, 9, 12, 90, 13] items=["10 u"=50, "100 u"=51, "1 m"=52, "10 m"=0, "20 m"=1, "50 m"=2, "100 m"=3, "200 m"=4, "500 m"=5, "1"=6, "2"=7, "3"=53, "5"=8, "10"=9, "20"=10, "50"=11, "100"=12, "700"=90, "1000"=13] ("Range [V]")
                      }
                    }
                    n100 = for {
                      tunnel: [w204] -> w199 mode=indexing if=w203
                      tunnel: w196 -> [w202]
                      tunnel: w195 -> [w201] mode=indexing
                      i -> [w204]
                      # "since DisabledItems works on the\nposition in the ring list, use the index\ni as output of this for loop"
                      n101 = Search 1D Array(1D array=w202, element=w201) -> (index of element=w206:i32)  [unwired: 1 in]
                      n102 = Equal?(x=-1, y=w206) -> (x = y?=w203:bool)
                    }
                    n103 = control-ref of="Range"() -> (w197:refnum<vi>)
                    n104 = control-ref of="Range"() -> (w198:refnum<vi>)
                    n105 = property class="Ring (strict)"(reference=w197, "Disabled Items []"=w199) -> ()  [unwired: 1 in, 2 out]
                    n106 = property class="Ring (strict)"(reference=w198, "Disabled Items []"=w199) -> ()  [unwired: 1 in, 2 out]
                  }
                }
              }
            }
            n107 = Wait (ms)(milliseconds to wait=u32 10) -> ()  [unwired: 1 out]
          }
        }
        frame #3 {
          n108 = case shown="True" TRUE {
            frame False {
            }
            frame True {
              n109 = invoke class="VI" method="FP.Close"() -> ()  [unwired: 3 in, 3 out]
            }
          }
        }
      }
      n110 = Unbundle By Name(w17) -> ("Hardware Configuration.Timing.Samples per Iteration"=→"Samples per Iteration":u32, "Hardware Configuration.Channel 1.Acquiring"=→"Acquiring":bool, "Hardware Configuration.Channel 2.Acquiring"=→"Acquiring":bool, "Hardware Configuration.Timing.Actual Sample Time [s]"=→"Actual Samping Time":dbl, "Hardware Configuration.DAQ Type"=w16:T11, "Logging Configuration.Log File Base Path"=w15:path)
      n111 = local write "Log File Path"(w15) -> ()
      n112 = local write "DAQ Type"(w16) -> ()
      n113 = case shown="False" w19 {
        tunnel: w18 -> [w213 _]
        frame False {
          # "Write settings back to XML"
          n114 = call "Get Config File Path.vi"() -> ("XML File Path"=w214:path)  [unwired: 10 in, 1 out]
          n115 = Flatten To XML(anything=w213) -> (xml string=w212:string)
          n116 = call-poly <vilib>:"Write to XML File.vi"("XML Input"=w212, "XML File Path"=w214) -> ()  [unwired: 7 in, 3 out]
        }
        frame True {
        }
      }
    }
    frame Error {
    }
  }
  "UI Refresh Needed?" <- w2
  "error out" <- w5
  "Settings out" <- w3
  "Cancelled?" <- w1
